vi "Test servers.vi"(9 "timeout ms (60000)":i32, 10 "port":u16, 11 "Server list":string[](array[string])) -> (2 "Server Stats":T1[](array[typedef]) {"channel settings"."lower input limits" format="%.4f"; "channel settings"."upper input limits" format="%.4f"; "scan rate" format="%.2f"}, 3 "Disabled items":i32[](array[numeric]))   [LabVIEW 2019]
uses:
  Process Controller 3.0/Distributed Daq/Daq cmd.ctl
  Server stats.ctl
panel:
  # "Hz"
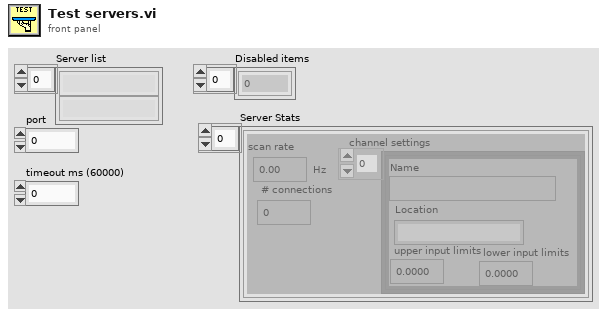
[diagram p1: front panel]
types:
  T1 = typedef "Server stats.ctl" = cluster{"scan rate":dbl, "# connections":i32, "channel settings":cluster{"Name":string, "upper input limits":sgl, "lower input limits":sgl, "Location":string}[]}
  T2 = typedef "Daq cmd.ctl" = enum16{"Start", "Get one scan", "Server Stats", "Stop Acquisition"}
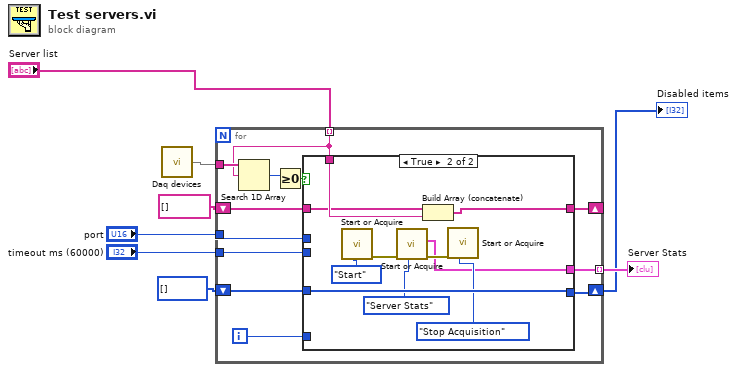
[diagram p0: block diagram]
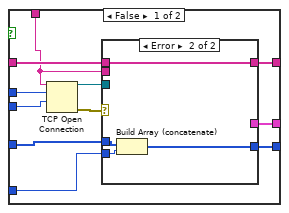
[diagram p2: hidden frame]
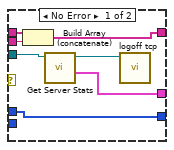
[diagram p3: hidden frame]
diagram:
  n1 = call "Daq devices.vi"() -> (4:w1)  [unwired: 5 in, 5 out]
  n2 = for {
    tunnel: "Server list" -> [w11] mode=indexing
    shift-right: [w20] -> _
    shift-left: string[] [] -> [w19]
    shift-right: [w17] -> w4
    shift-left: i32[] [] -> [w16]
    tunnel: "port" -> [w15]
    tunnel: "timeout ms (60000)" -> [w14]
    tunnel: [w13] -> w7 mode=indexing
    tunnel: w1 -> [w12]
    i -> [w18]
    n3 = Search 1D Array(1D array=w12, element=w11) -> (index of element=w10:i32)  [unwired: 1 in]
    n4 = Greater Or Equal To 0?(x=w10) -> (x >= 0?=w9:bool)
    n5 = case shown="True" w9 {
      tunnel: [w30 w49] -> w20
      tunnel: w19 -> [w29 w51]
      tunnel: w18 -> [w28 _]
      tunnel: [w27 w50] -> w17
      tunnel: w16 -> [w26 w50]
      tunnel: w15 -> [w24 _]
      tunnel: w14 -> [w23 _]
      tunnel: [w22 w43] -> w13
      tunnel: w11 -> [w21 w52]
      frame False {
        n6 = TCP Open Connection(address=w21, remote port or service name=w24, timeout ms (60000)=w23) -> (connection ID=w25:refnum<k5>, error out=w31:errorcluster)  [unwired: 2 in]
        n7 = case shown="Error" w31 {
          tunnel: w21 -> [w38 _]
          tunnel: [w37 w42] -> w30
          tunnel: w29 -> [w36 w42]
          tunnel: w28 -> [_ w41]
          tunnel: [w35 w40] -> w27
          tunnel: w26 -> [w35 w39]
          tunnel: w25 -> [w34 _]
          tunnel: [w32 _] -> w22
          frame No Error {
            n8 = Build Array (concatenate)(w36, w38) -> (w37:string[])
            n9 = call "Get Server Stats.vi"("Connection ID"=w34) -> ("Server stats"=w32:T1, "Connection ID"=w33:refnum<k5>)  [unwired: 7 in, 2 out]
            n10 = call "logoff tcp.vi"("Connection ID"=w33) -> ()  [unwired: 9 in, 2 out]
          }
          frame Error {
            n11 = Build Array (concatenate)(w39, w41) -> (w40:i32[])
          }
        }
      }
      frame True {
        n12 = call "Start or Acquire.vi"("Daq cmd"=Daq_cmd."Start") -> ("error out"=w48:errorcluster)  [unwired: 8 in, 2 out]
        n13 = call "Start or Acquire.vi"("Daq cmd"=Daq_cmd."Server Stats", "error in (no error)"=w48) -> ("error out"=w47:errorcluster, "Server Stats"=w43:T1)  [unwired: 7 in, 1 out]
        n14 = Build Array (concatenate)(w51, w52) -> (w49:string[])
        n15 = call "Start or Acquire.vi"("Daq cmd"=Daq_cmd."Stop Acquisition", "error in (no error)"=w47) -> ()  [unwired: 7 in, 3 out]
      }
    }
  }
  "Server Stats" <- w7
  "Disabled items" <- w4
